vi "file_path.vi"(10 "name identifier":string, 11 "Base path":path=path "C:/Users/MPI/Desktop") -> (0 "HDF path":path, 1 "TDMS time domain path":path, 4 "TDMS path":path)   [LabVIEW 2021]
panel:
  out "OnlineReconPath":path
  # "Used when storing in HDF format"
  # "Used when storing time domain"
  # "Used when storing in TDMS format"
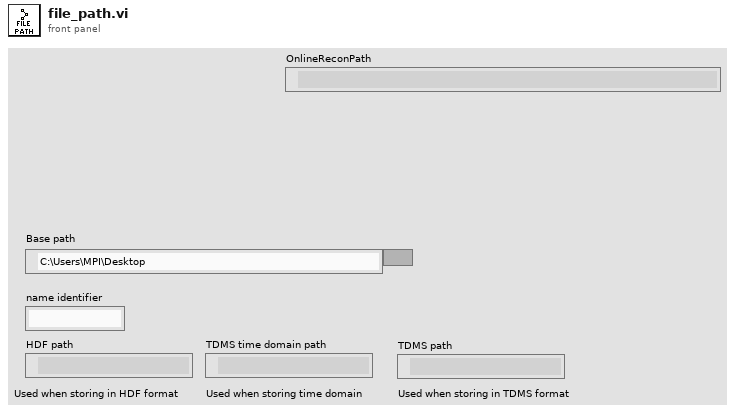
[diagram p1: front panel]
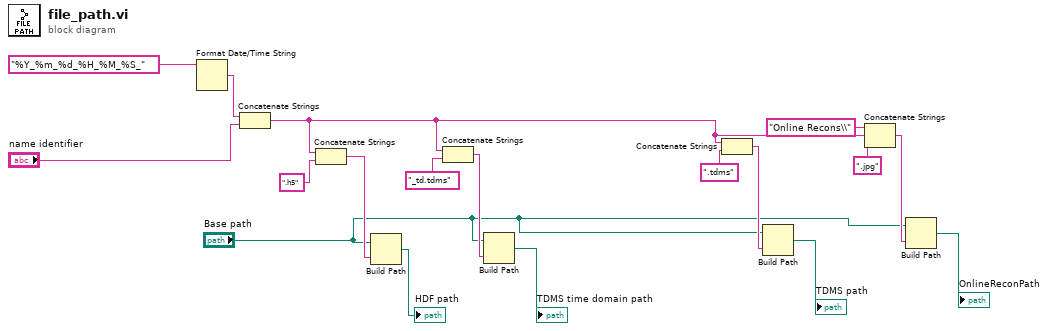
[diagram p0: block diagram]
diagram:
  n1 = Format Date/Time String(time format string (%c)="%Y_%m_%d_%H_%M_%S_") -> (date/time string=w18:string)  [unwired: 2 in]
  n2 = Concatenate Strings(w18, "name identifier") -> (w2:string)
  n3 = Concatenate Strings(w2, ".h5" ("string")) -> (w14:string)
  n4 = Build Path(base path="Base path", name or relative path=w14) -> (appended path=→"HDF path":path)
  n5 = Concatenate Strings(w2, "_td.tdms" ("string")) -> (w12:string)
  n6 = Build Path(base path="Base path", name or relative path=w12) -> (appended path=→"TDMS time domain path":path)
  n7 = Concatenate Strings(w2, ".tdms" ("string")) -> (w8:string)
  n8 = Build Path(base path="Base path", name or relative path=w8) -> (appended path=→"TDMS path":path)
  n9 = Concatenate Strings("Online Recons\\" ("string"), w2, ".jpg" ("string")) -> (w5:string)
  n10 = Build Path(base path="Base path", name or relative path=w5) -> (appended path=→"OnlineReconPath":path)
